vi "Update Control States.vi"(8 "error in (no error)":errorcluster, 10 "ATM State":T1, 11 "ATM View Model In":refnum<class "ATM View Model.lvclass">) -> (0 "error out":errorcluster, 3 "ATM View Model Out":refnum<class "ATM View Model.lvclass">)   [LabVIEW 2020, in "ATM View Model.lvclass"]
uses:
  ATM View Model.lvclass
  ATM Controller/State.ctl
  ATM Controller/ATM Controller.lvclass
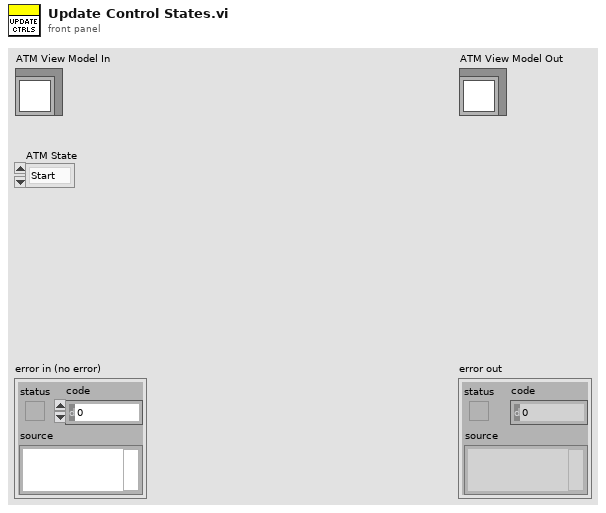
[diagram p1: front panel]
types:
  T1 = typedef "ATM Controller.lvclass/State.ctl" = enum16{"Start", "Card Inserted", "Verification Failed", "Verification Succeeded", "Depositing", "Depositing Completed", "Withdrawing", "Withdraw Completed", "Withdraw Failed", "Balance Inquiry", "Terminate"}
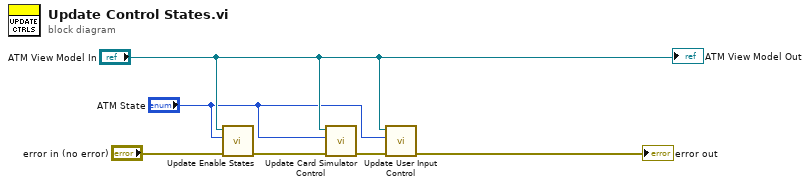
[diagram p0: block diagram]
diagram:
  n1 = call "Update Enable States.vi"("error in (no error)"="error in (no error)", "ATM State"="ATM State", "ATM View Model in"="ATM View Model In") -> ("error out"=w5:errorcluster)  [unwired: 8 in]
  n2 = call "Update Card Simulator Control.vi"("error in (no error)"=w5, "ATM State"="ATM State", "ATM View Model in"="ATM View Model In") -> ("error out"=w3:errorcluster)  [unwired: 8 in]
  n3 = call "Update User Input Control.vi"("error in (no error)"=w3, "ATM State"="ATM State", "ATM View Model in"="ATM View Model In") -> ("error out"=→"error out":errorcluster)  [unwired: 8 in]
  "ATM View Model Out" <- "ATM View Model In"
